vi "Get System Channels Info.vi"(8 "error in (no error)":errorcluster, 11 "Item Ref in":T1 format="%.0x") -> (0 "error out":errorcluster, 1 "Channel Names":string[](array[string]), 2 "Channel Refs":T1[](array[typedef]) format="%.0x", 3 "Item Ref out":T1 format="%.0x", 4 "Channel Paths":string[](array[string]))   [LabVIEW 2019, in "Telemetry Engine.lvlib"]
uses:
  <vilib>/NI VeriStand/Custom Device API/Custom Device Item Ref.ctl
  Shared/Constants.vi
  <vilib>/NI VeriStand/Custom Device API/Set Item Property (String Array).vi
  Engine/Telemetry Engine.lvlib
  <vilib>/NI VeriStand/Custom Device Tools/Custom Device Utility Library/Custom Device Utility Library.lvlib
  <vilib>/NI VeriStand/Custom Device API/Custom Device API.lvlib
  Shared/Telemetry Shared.lvlib
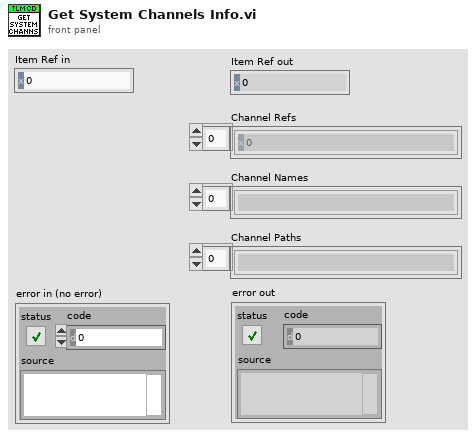
[diagram p1: front panel]
types:
  T1 = typedef "Custom Device API.lvlib/Custom Device Item Ref.ctl" = u64
  T2 = typedef "Custom Device API.lvlib/Custom Device Item Info.ctl" = cluster{"Name":string, "Is Channel":bool, "GUID":string, "Is Waveform":bool}
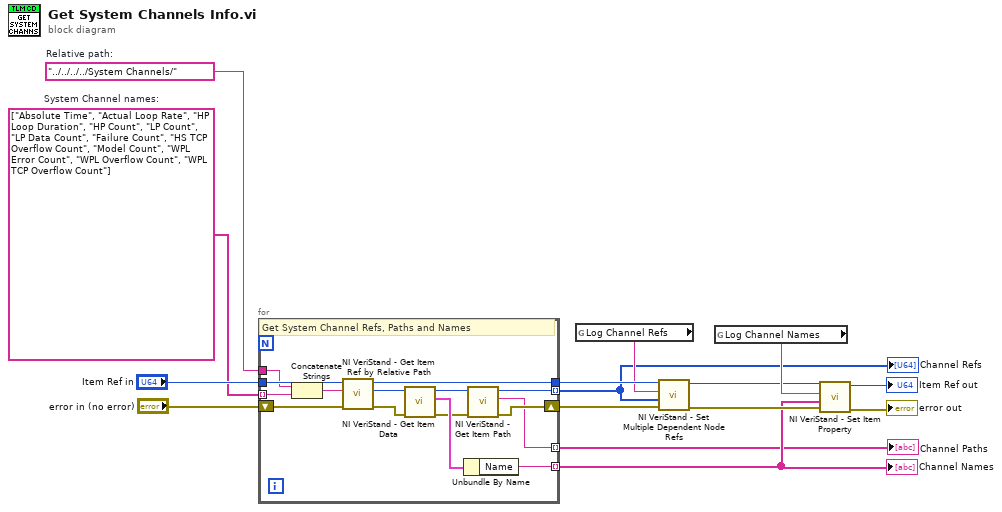
[diagram p0: block diagram]
diagram:
  w1 = "../../../../System Channels/"  # Relative path:
  w2 = string[] ["Absolute Time", "Actual Loop Rate", "HP Loop Duration", "HP Count", "LP Count", "LP Data Count", "Failure Count", "HS TCP Overflow Count", "Model Count", "WPL Error Count", "WPL Overflow Count", "WPL TCP Overflow Count"]  # System Channel names:
  n1 = for {
    tunnel: "Item Ref in" -> [w30]
    shift-right: [w22] -> w14
    shift-left: "error in (no error)" -> [w29]
    tunnel: [w21] -> w10
    tunnel: [w20] -> w6 mode=indexing
    tunnel: [w25] -> w7 mode=indexing
    tunnel: [w19] -> w4 mode=indexing
    tunnel: w2 -> [w17] mode=indexing
    tunnel: w1 -> [w16]
    # "Get System Channel Refs, Paths and Names"
    n2 = Concatenate Strings(w16, w17) -> (w18:string)
    n3 = call <vilib>:"NI VeriStand - Get Item Ref by Relative Path.vi"("error in"=w29, "Relative Item Path"=w18, "Section Ref in"=w30) -> ("error out"=w28:errorcluster, "Item Ref"=w27:T1, "Section Ref out"=w21:T1)  [unwired: 5 in, 1 out]
    n4 = call <vilib>:"NI VeriStand - Get Item Data.vi"("error in (no error)"=w28, "Item Ref in"=w27) -> ("error out"=w23:errorcluster, "Item Info"=w26:T2, "Item Ref out"=w24:T1)  [unwired: 6 in, 1 out]
    n5 = Unbundle By Name(w26) -> ("Name"=w25:string)
    n6 = call <vilib>:"NI VeriStand - Get Item Path.vi"("error in (no error)"=w23, "Item Ref in"=w24) -> ("error out"=w22:errorcluster, "Path"=w19:string, "Item Ref out"=w20:T1)  [unwired: 6 in, 1 out]
  }
  "Channel Names" <- w7
  "Channel Refs" <- w6
  "Channel Paths" <- w4
  n7 = global read "Constants.vi" "Log Channel Refs"() -> (w8:string)
  n8 = call <vilib>:"NI VeriStand - Set Multiple Dependent Node Refs.vi"("error in (no error)"=w14, "Dependent Node Refs"=w6, "Base Property Name"=w8, "Item Ref in"=w10) -> ("error out"=w13:errorcluster, "Item Ref out"=w9:T1)  [unwired: 6 in]
  n9 = global read "Constants.vi" "Log Channel Names"() -> (w11:string)
  n10 = call-poly <vilib>:"NI VeriStand - Set Item Property.vi"("error in (no error)"=w13, "Value"=w7, "Property Name"=w11, "Item Ref in"=w9) -> ("error out"=→"error out":errorcluster, "Item Ref out"=→"Item Ref out":T1)  [unwired: 5 in, 1 out]
